vi "Save State.vi"(8 "error in":errorcluster, 9 "Out-of-range List":string[](array[string]), 10 "Monitoring List":string[](array[string]), 11 "State File Refnum in":refnum<file>) -> (0 "error out":errorcluster, 3 "State File Refnum out":refnum<file>)   [LabVIEW 2013, in "ACNET Monitor.lvlib"]
uses:
  ACNET Monitor.lvlib
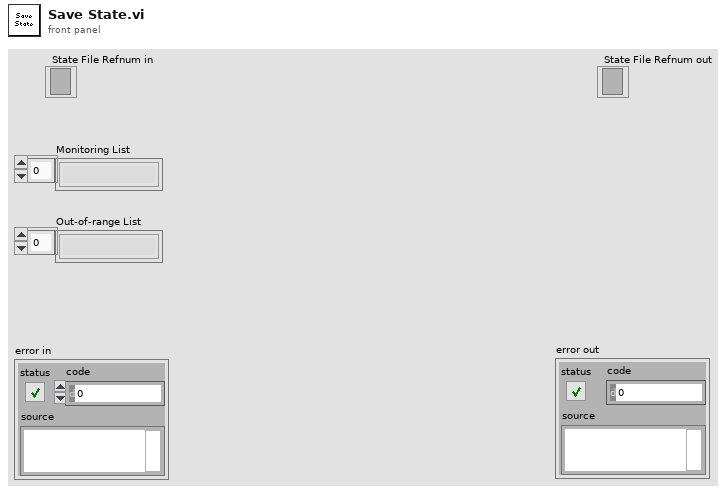
[diagram p1: front panel]
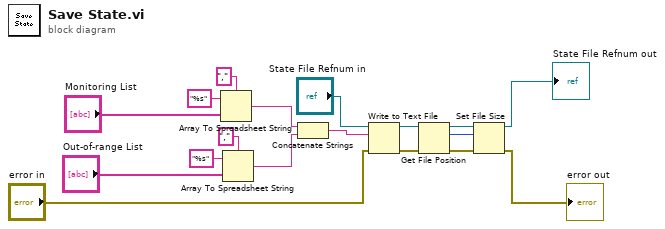
[diagram p0: block diagram]
diagram:
  n1 = Array To Spreadsheet String(delimiter (Tab)=",", array="Monitoring List", 3:"%s" ("format string")) -> (spreadsheet string=w11:string)
  n2 = Array To Spreadsheet String(delimiter (Tab)=",", array="Out-of-range List", 3:"%s" ("format string")) -> (spreadsheet string=w10:string)
  n3 = Concatenate Strings(w11, w10) -> (w9:string)
  n4 = Write to Text File(file (use dialog)="State File Refnum in", text=w9, error in="error in") -> (refnum out=w4:refnum<file>, error out=w5:errorcluster)  [unwired: 1 in, 1 out]
  n5 = Get File Position(4:w5, 7:w4) -> (0:w7:errorcluster, 2:w6:i64, 3:w2:refnum<file>)
  n6 = Set File Size(4:w7, 6:w6, 7:w2) -> (0:→"error out":errorcluster, 3:→"State File Refnum out":refnum<file>)
